vi "moco_for_sub.vi"(0 "Communication port":refnum<visa-resource-name>="COM1", 1 "Destination Wavelength":dbl=500.0 format="%.2f", 2 "GoTo":bool, 3 "Wavelength, nm":dbl=10.0 format="%.2f", 4 "bs":bool, 5 "fs":bool, 6 "Sh_ON":bool, 7 "Sh_OFF":bool) -> (20 "read string":string="\n", 21 "Present Wavelength":dbl format="%.2f", 22 "Suuter":bool)   [LabVIEW 2018]
doc: "Monochromator control"
uses:
  global_m.vi
panel:
  in  "Start up Blinking":bool=TRUE
  in  "Delay Before\nread (ms)":u32=50
  out "dalay":u16
  out "button":i32
  out "back_L":bool
  out "Shutter OFF":bool
  out "Shutter ON":bool
  in  "Tab Control":enum32{"Setup", "Operation"}(tab)
  in  "Save settings":bool
  in  "Initialize":bool caption="Push at start up"
  in  "Grating, gr/mm":u16(ring)=2 items=["2400", "1800", "1200", "600", "300", "150"]
  in  "Backlash compensation":dbl=10.0 format="%.2f"
  in  "Backlash":bool
  in  "Calibration, nm":dbl=265.0 format="%2.2f"
  in  "Speed_set":bool
  in  "Speed":dbl=50.0 format="%.3f"
  in  "stop 2":bool
  out "move done":bool
  out "string 2":string="\n"
  in  "return":bool
  in  "String To Write 3":string="Y-1?"
  out "Loop":i32
  in  "write":bool
  out "command sent":string="\n"
  out "writing":bool
  in  "stop":bool
  # "Backlash \nCompensation, nm"
  # "nm"
  # "Wavelength"
  # "nm"
  # "Move Wavelength"
  # "nm"
  # "nm/sec"
  # "Shutter"
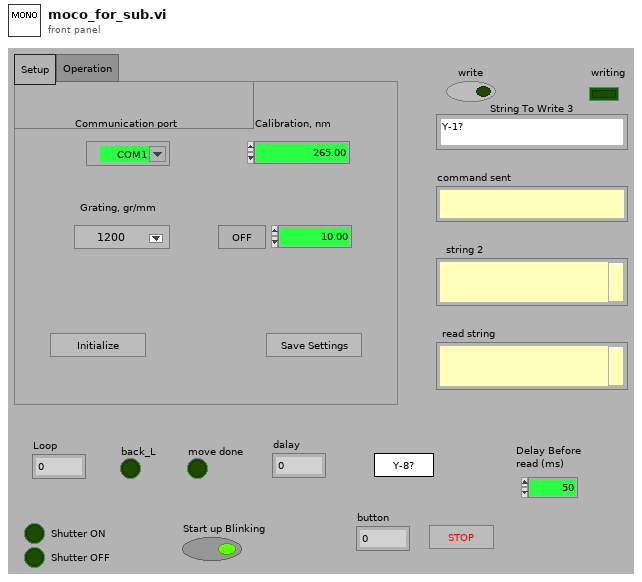
[diagram p1: front panel]
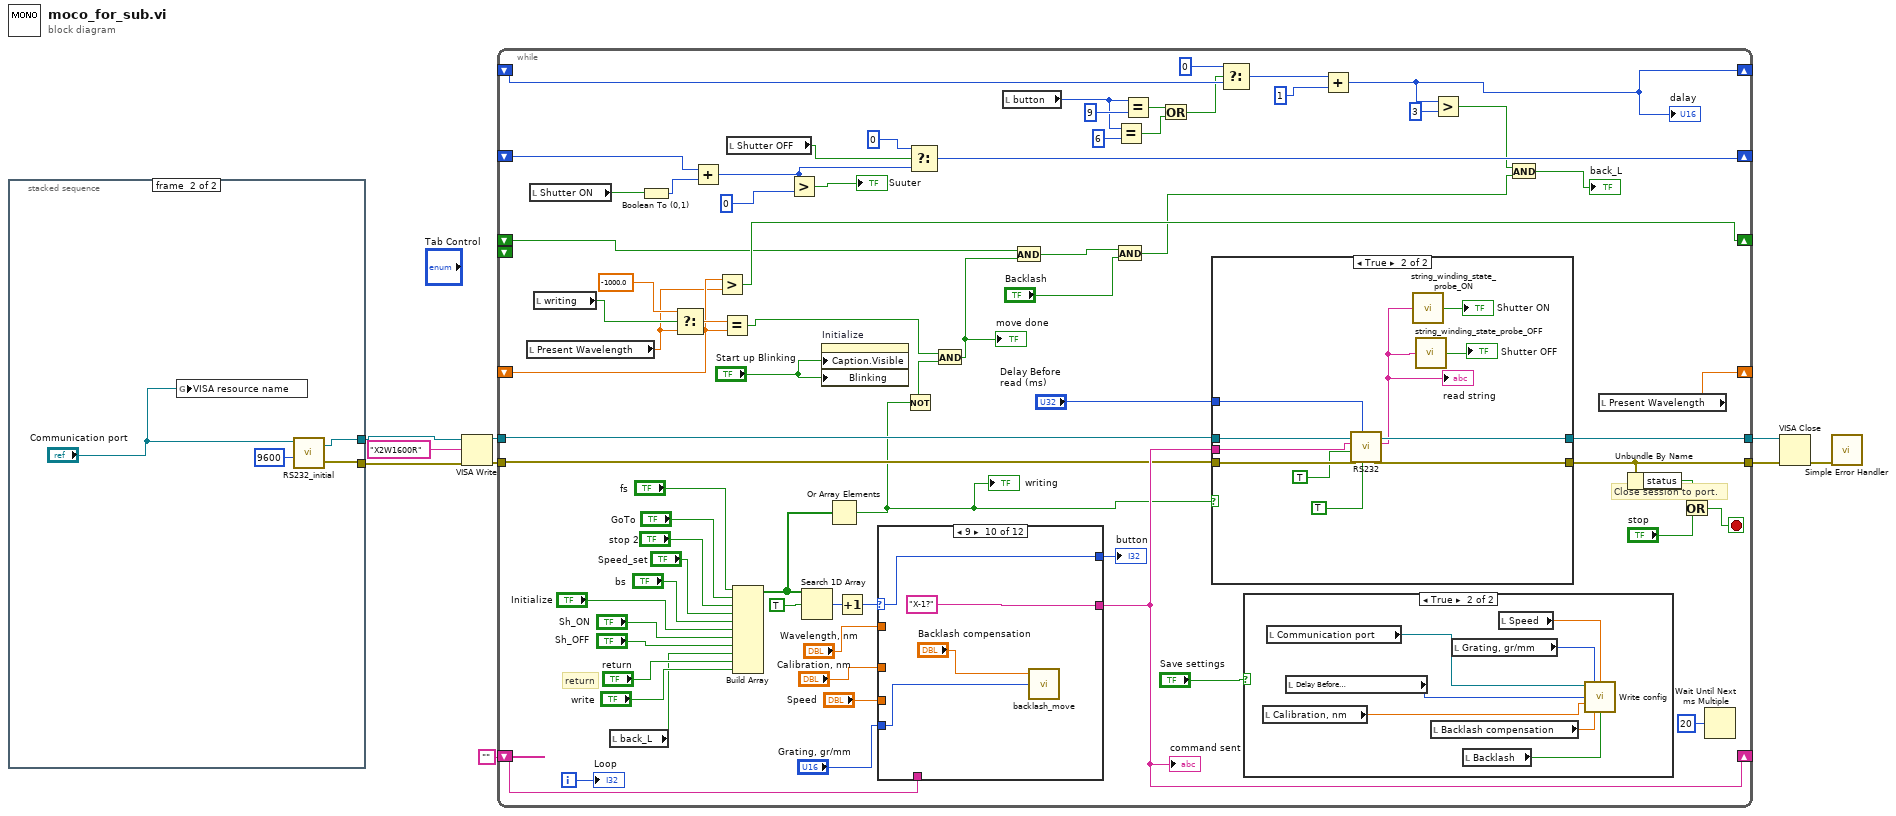
[diagram p0: block diagram]
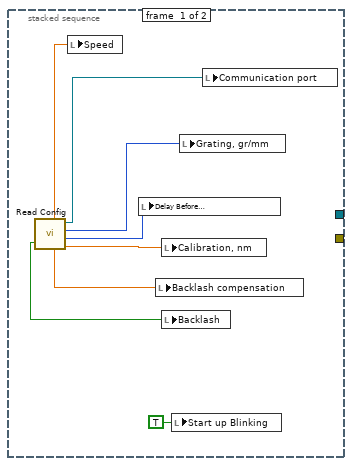
[diagram p2: hidden frame]
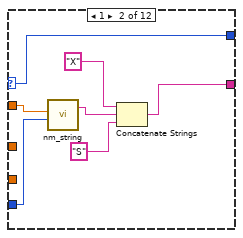
[diagram p5: hidden frame]
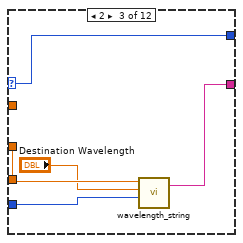
[diagram p6: hidden frame]
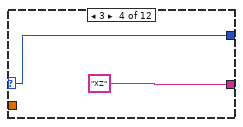
[diagram p7: hidden frame]
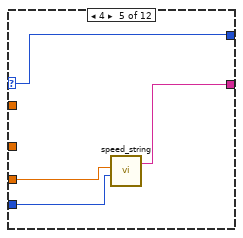
[diagram p8: hidden frame]
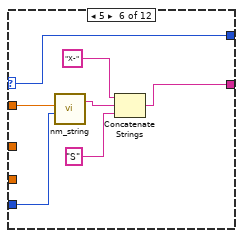
[diagram p9: hidden frame]
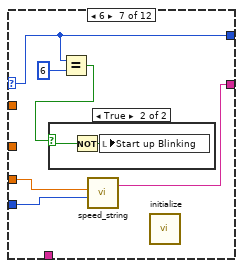
[diagram p10: hidden frame]
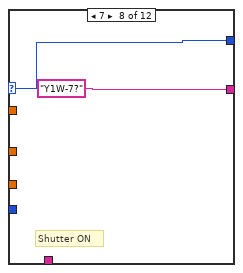
[diagram p12: hidden frame]
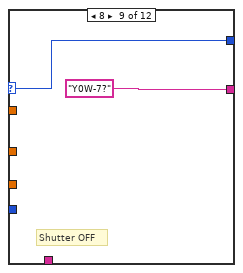
[diagram p13: hidden frame]
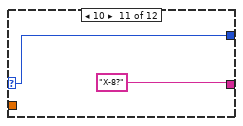
[diagram p14: hidden frame]
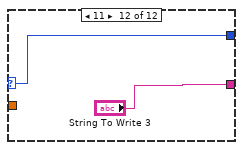
[diagram p15: hidden frame]
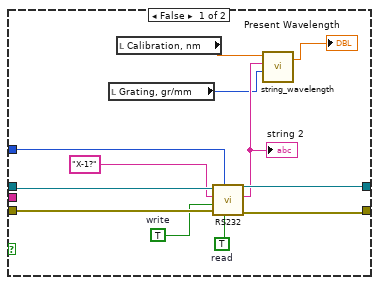
[diagram p16: hidden frame]
diagram:
  n1 = stacked-sequence {
    tunnel: [_ w21] -> w2
    tunnel: [_ w20] -> w1
    frame #0 {
      n2 = call "Read Config.vi"() -> ("Backlash"=w14:bool, "Speed"=w17:dbl, "Backlash compensation"=w15:dbl, "VISA resource name"=w12:refnum<visa-resource-name>, "Grating, gr/mm"=w13:u16, "Delay Before read (ms)"=w11:u32, "Calibration, nm"=w16:dbl)  [unwired: 1 in]
      n3 = local write "Speed"(w17) -> ()
      n4 = local write "Delay Before\nread (ms)"(w11) -> ()
      n5 = local write "Backlash compensation"(w15) -> ()
      n6 = local write "Calibration, nm"(w16) -> ()
      n7 = local write "Backlash"(w14) -> ()
      n8 = local write "Start up Blinking"(TRUE ("Start up Blinking")) -> ()
      n9 = local write "Grating, gr/mm"(w13) -> ()
      n10 = local write "Communication port"(w12) -> ()
    }
    frame #1 {
      n11 = global write "global_m.vi" "VISA resource name"("Communication port") -> ()
      n12 = call "RS232_initial.vi"("baud rate"=u32 9600, "VISA resource name"="Communication port") -> ("error out"=w20:errorcluster, "VISA name out"=w21:refnum<visa-resource-name>)  [unwired: 2 in]
    }
  }
  n13 = VISA Write(VISA resource name=w2, write buffer="X2W1600R", error in (no error)=w1) -> (VISA resource name out=w5:refnum<visa-resource-name>, error out=w4:errorcluster)  [unwired: 1 out]
  n14 = while {
    tunnel: [w93] -> w8
    tunnel: [w92] -> w7
    tunnel: w5 -> [w80]
    tunnel: w4 -> [w79]
    shift-right: [w81] -> _
    shift-left: "" -> [w84]
    shift-right: [w67] -> _
    shift-left: _ -> [w48]
    shift-right: [w50] -> _
    shift-left: _ -> [w56]
    shift-right: [w46] -> _
    shift-left: _ -> [w45]
    shift-left: _ -> [_]
    shift-right: [w30] -> _
    shift-left: _ -> [w41]
    i -> [w82]
    stop <- w89 stop-if-true
    # "return"
    # "Close session to port."
    n15 = local read "Present Wavelength"() -> (w47:dbl)
    n16 = local read "Shutter ON"() -> (w58:bool)
    n17 = local read "writing"() -> (w62:bool)
    n18 = local read "back_L"() -> (w39:bool)
    n19 = Boolean To (0,1)(Boolean=w58) -> (0, 1=w57:i16)
    n20 = Select(t=-1000.0 ("f"), s=w62, f=w47) -> (s? t:f=w63:dbl)
    n21 = Add(x=w56, y=w57) -> (x+y=w53:i16)
    n22 = Greater?(x=w48, y=w47) -> (0:w46:bool)
    n23 = Equal?(x=w63, y=w48) -> (x = y?=w64:bool)
    n24 = local read "Shutter OFF"() -> (w52:bool)
    n25 = Build Array "Build Array"("fs", "GoTo", "stop 2", "Speed_set", "bs", "Initialize", "Sh_ON", "Sh_OFF", w39, "return", "write") -> (w83:bool[])
    n26 = Greater?(x=w53, y=i16 0) -> (0:→"Suuter":bool)
    n27 = Search 1D Array(1D array=w83, element=TRUE) -> (index of element=w86:i32)  [unwired: 1 in]
    n28 = property on="Initialize" class="Bool"("Caption.Visible"="Start up Blinking", "Blinking"="Start up Blinking") -> ()  [unwired: 2 in, 2 out]
    n29 = Or Array Elements(Boolean array=w83) -> (logical OR=w66:bool)
    "writing" <- w66
    n30 = Increment(x=w86) -> (x+1=w85:i32)
    n31 = case shown="9" w85 {
      selector: w85 -> [w101 w109 w114 w116 w120 w127 w130 w137 w139 w143 w145 w146]
      tunnel: [w102 w106 w111 "XZ" ("string to write 2") w119 w124 w131 "Y1W-7?" ("string") "Y0W-7?" "X-1?" "X-8?" "String To Write 3"] -> w81
      tunnel: w84 -> [w102 _ _ _ _ _ _ _ _ _ _ _]
      tunnel: [w101 w109 w114 w116 w120 w127 w130 w137 w139 w143 w145 w146] -> w43
      tunnel: "Wavelength, nm" -> [_ w105 _ _ _ w123 _ _ _ _ _ _]
      tunnel: "Calibration, nm" -> [_ _ w113 _ _ _ _ _ _ _ _ _]
      tunnel: "Grating, gr/mm" -> [_ w104 w112 _ w117 w122 w132 _ _ w141 _ _]
      tunnel: "Speed" -> [_ _ _ _ w118 _ w133 _ _ _ _ _]
      frame ..0, Default {
        # "no change"
      }
      frame 1 {
        n32 = call "nm_string.vi"("Grating, gr/mm"=w104, "Wavelength, nm"=w105) -> ("nm_String"=w103:string)  [unwired: 2 in, 1 out]
        n33 = Concatenate Strings("X" ("string"), w103, "S" ("string")) -> (w106:string)
      }
      frame 2 {
        n34 = call "wavelength_string.vi"("Grating, gr/mm"=w112, "Destination Wavelength"="Destination Wavelength", "Calibration, nm"=w113) -> ("Wavelength_String"=w111:string)  [unwired: 1 in, 1 out]
      }
      frame 3 {
      }
      frame 4 {
        n35 = call "speed_string.vi"("Grating, gr/mm"=w117, "Speed"=w118) -> ("nm_String"=w119:string)  [unwired: 2 in, 1 out]
      }
      frame 5 {
        n36 = call "nm_string.vi"("Grating, gr/mm"=w122, "Wavelength, nm"=w123) -> ("nm_String"=w121:string)  [unwired: 2 in, 1 out]
        n37 = Concatenate Strings("X-" ("string"), w121, "S" ("string")) -> (w124:string)
      }
      frame 6 {
        n38 = Equal?(x=w130, y=6) -> (x = y?=w128:bool)
        n39 = case shown="True" w128 {
          selector: w128 -> [_ w134]
          frame False {
          }
          frame True {
            n40 = Not(x=w134) -> (.not. x?=w135:bool)
            n41 = local write "Start up Blinking"(w135) -> ()
          }
        }
        n42 = call "speed_string.vi"("Grating, gr/mm"=w132, "Speed"=w133) -> ("nm_String"=w131:string)  [unwired: 2 in, 1 out]
        n43 = call "initialize.vi"() -> ()  [unwired: 3 in]
      }
      frame 7 {
        # "Shutter ON"
      }
      frame 8 {
        # "Shutter OFF"
      }
      frame 9 {
        n44 = call "backlash_move.vi"("Grating, gr/mm"=w141, "Wavelength, nm"="Backlash compensation") -> ()  [unwired: 3 in]
      }
      frame 10 {
      }
      frame 11 {
      }
    }
    "command sent" <- w81
    "button" <- w43
    n45 = Not(x=w66) -> (.not. x?=w65:bool)
    n46 = Select(t=i16 0, s=w52, f=w53) -> (s? t:f=w50:i16)
    n47 = And(x=w64, y=w65) -> (x .and. y?=w44:bool)
    "move done" <- w44
    n48 = local read "button"() -> (w34:i32)
    n49 = And(x=w45, y=w44) -> (x .and. y?=w38:bool)
    n50 = And(x=w38, y="Backlash") -> (x .and. y?=w28:bool)
    n51 = Equal?(x=w34, y=6) -> (x = y?=w35:bool)
    n52 = Equal?(x=w34, y=9) -> (x = y?=w37:bool)
    n53 = Or(x=w37, y=w35) -> (x .or. y?=w36:bool)
    n54 = case shown="True" w66 {
      tunnel: [w159 w166] -> w93
      tunnel: [w156 w165] -> w92
      tunnel: w80 -> [w158 w170]
      tunnel: w79 -> [w157 w168]
      tunnel: w81 -> [_ w169]
      tunnel: "Delay Before\nread (ms)" -> [w148 w167]
      frame False {
        w153 = TRUE  # read
        w154 = TRUE  # write
        n55 = local read "Grating, gr/mm"() -> (w149:u16)
        n56 = local read "Calibration, nm"() -> (w150:dbl)
        n57 = call "RS232.vi"("read"=w153, "delay before read (ms)"=w148, "error in"=w157, "write"=w154, "string to write"="X-1?", "VISA  name in"=w158) -> ("error out"=w156:errorcluster, "read string"=w151:string, "VISA out"=w159:refnum<visa-resource-name>)  [unwired: 1 out]
        "string 2" <- w151
        n58 = call "string_wavelength.vi"("Grating, gr/mm"=w149, "Position String"=w151, "Calibration, nm"=w150) -> ("Present Wavelength"=→"Present Wavelength":dbl)  [unwired: 1 in, 1 out]
      }
      frame True {
        n59 = call "RS232.vi"("read"=TRUE, "delay before read (ms)"=w167, "error in"=w168, "write"=TRUE, "string to write"=w169, "VISA  name in"=w170) -> ("error out"=w165:errorcluster, "read string"=w162:string, "VISA out"=w166:refnum<visa-resource-name>)  [unwired: 1 out]
        "read string" <- w162
        n60 = call "string_winding_state_probe_ON.vi"("read string"=w162) -> ("ON"=→"Shutter ON":bool)
        n61 = call "string_winding_state_probe_OFF.vi"("read string"=w162) -> ("OFF"=→"Shutter OFF":bool)
      }
    }
    n62 = Select(t=u16 0, s=w36, f=w41) -> (s? t:f=w32:u16)
    n63 = case shown="True" "Save settings" {
      frame False {
      }
      frame True {
        n64 = local read "Calibration, nm"() -> (w100:dbl)
        n65 = local read "Communication port"() -> (w94:refnum<visa-resource-name>)
        n66 = local read "Delay Before\nread (ms)"() -> (w95:u32)
        n67 = local read "Backlash compensation"() -> (w97:dbl)
        n68 = local read "Grating, gr/mm"() -> (w96:u16)
        n69 = local read "Backlash"() -> (w98:bool)
        n70 = local read "Speed"() -> (w99:dbl)
        n71 = call "Write config.vi"("VISA resource name"=w94, "Grating, gr/mm"=w96, "Speed"=w99, "Delay Before read (ms)"=w95, "Calibration, nm"=w100, "Backlash compensation"=w97, "Backlash"=w98) -> ()  [unwired: 9 in]
      }
    }
    n72 = Add(x=w32, y=u16 1) -> (x+y=w30:u16)
    "dalay" <- w30
    n73 = Greater?(x=w30, y=u16 3) -> (0:w27:bool)
    n74 = And(x=w27, y=w28) -> (x .and. y?=→"back_L":bool)
    n75 = local read "Present Wavelength"() -> (w67:dbl)
    n76 = Unbundle By Name(w92) -> ("status"=w91:bool)
    n77 = Or(x=w91, y="stop") -> (x .or. y?=w89:bool)
    n78 = Wait Until Next ms Multiple(millisecond multiple=u32 20) -> ()  [unwired: 1 out]
    "Loop" <- w82
  }
  n79 = VISA Close(VISA resource name=w8, error in (no error)=w7) -> (error out=w9:errorcluster)
  n80 = call <vilib>:"Simple Error Handler.vi"("error in (no error)"=w9) -> ()  [unwired: 4 in, 5 out]
